vi "Handle M24.vi"(0 "reference in":refnum<class "PM_Group.lvclass">, 11 "error in (no error)":errorcluster) -> (4 "reference out":refnum<class "PM_Group.lvclass">, 15 "error out":errorcluster)   [LabVIEW 2019, in "PM_Group.lvclass"]
uses:
  PM_Group.lvclass
  C:/Users/ANENKOV_V1/Desktop/src/Device_class/Device.lvclass
  PM_Group.lvclass/PM_Group.ctl
  FPGA/TypeDef/AI index.ctl
  TypeDef/State Engine.ctl
  AI_class/AI.lvclass/AI.ctl
  AnalogComparator_class/AnalogComparator.lvclass/AnalogComparator.ctl
  Device_class/Device.lvclass/Device.ctl
  Engine_1DO_2DI_class/Engine_1DO_2DI.lvclass/Engine_1DO_2DI.ctl
  FPGA/TypeDef/DO index.ctl
  AnalogComparator_class/GetStatus.vi
  Engine_1DO_2DI_class/Engine_1DO_2DI.lvclass
  FPGA_API_class/FPGA API.lvclass
  AI_class/AI.lvclass
  Device_class/Device.lvclass
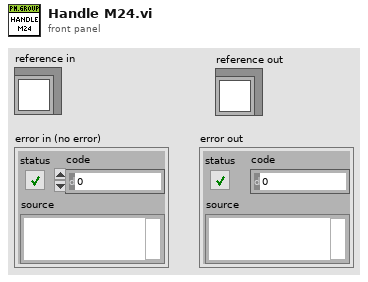
[diagram p1: front panel]
types:
  T1 = typedef "State Engine.ctl" = enum16{"Unknown", "Off", "TupningOn", "On", "TurningOff"}
  T2 = typedef "AI index.ctl" = u8
  T3 = typedef "AI_Data.ctl" = cluster{"Stat Data":T4, "OutOfRangeMax":bool, "OutOfRangeMin":bool, "HIHI":bool, "HI":bool, "LO":bool, "LOLO":bool}
  T4 = typedef "AI Statistics Data.ctl" = cluster{"raw mean":dbl, "scl mean":dbl, "raw mean 1Hz":dbl, "scl mean 1Hz":dbl}
  T5 = typedef "DO index.ctl" = u8
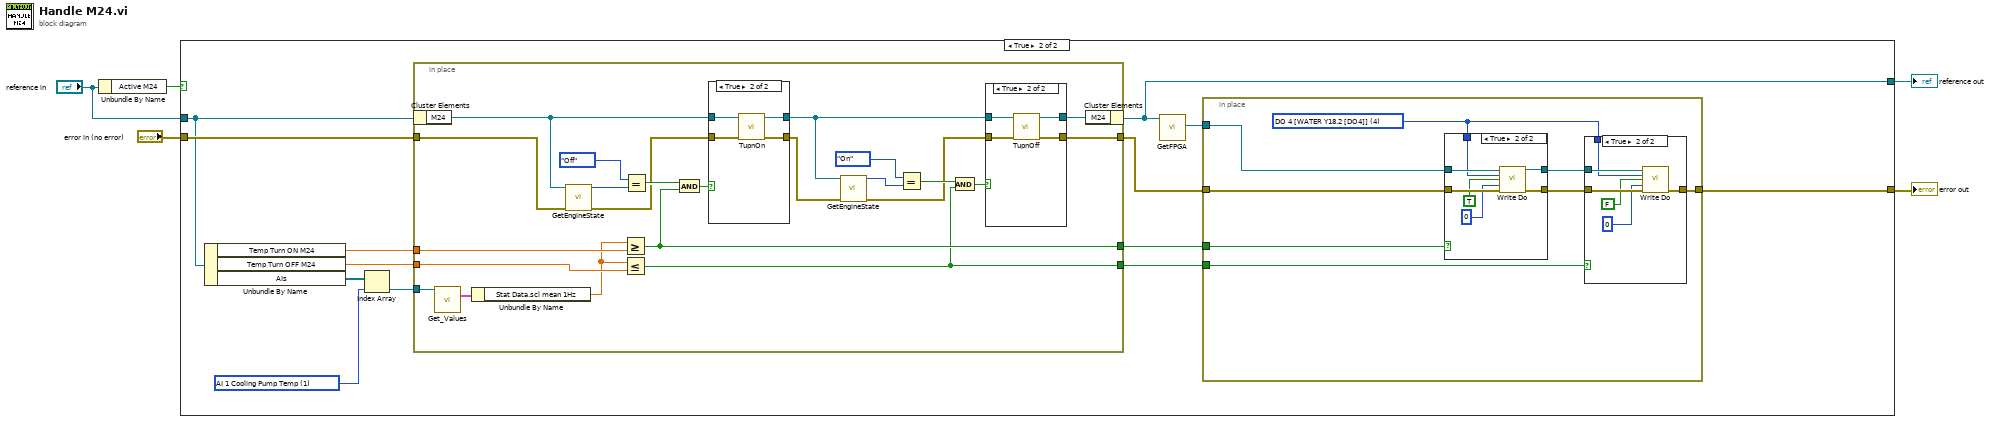
[diagram p0: block diagram]
diagram:
  n1 = Unbundle By Name("reference in") -> ("Active M24"=w1:bool)
  n2 = case shown="True" w1 {
    tunnel: "error in (no error)" -> [w6 w20]
    tunnel: "reference in" -> [w7 w14]
    tunnel: [w6 w16] -> w4
    tunnel: [w7 w15] -> w3
    frame False {
    }
    frame True {
      w10 = T2 1 items=["AI 0 Cooling Pump Level", "AI 1 Cooling Pump Temp", "AI 2 Oil Supply Level", "AI 3 Oil Supply Temp", "AI 4 ", "AI 5 Pressure Haskel", "AI 6 Pressure DUT", "AI 7 Pressure Chamber", "AI 8 Pressure Air inlet", "AI 9 Pressure Air outlet", "AI 10 Pressure Messure Line"] ("AI index")
      n3 = Unbundle By Name(w14) -> ("Temp Turn ON M24"=w13:dbl, "Temp Turn OFF M24"=w12:dbl, "AIs"=w11:refnum<class "AI.lvclass">[])
      n4 = Index Array(array=w11, index=w10) -> (element=w19:refnum<class "AI.lvclass">)
      n5 = in-place {
        in-place-border: w13 -> [w53]
        in-place-border: w12 -> [w54]
        in-place-border: w19 -> [w67]
        in-place-border: w20 -> [w50]
        in-place-border: [w59] -> w17
        in-place-border: [w46] -> w9
        in-place-border: [w45] -> w8
        n6 = in-place-cluster #1(w14) -> ("M24"=w65:refnum<class "Engine_1DO_2DI.lvclass">)
        n7 = call "Get_Values.vi"("reference in"=w67) -> ("Data"=w66:T3)  [unwired: 14 in]
        n8 = Unbundle By Name(w66) -> ("Stat Data.scl mean 1Hz"=w51:dbl)
        n9 = call "GetEngineState.vi"("Engine"=w65, "error in (no error)"=w50) -> ("EngineState"=w64:T1, "error out"=w49:errorcluster)  [unwired: 9 in, 3 out]
        n10 = Greater Or Equal?(x=w51, y=w53) -> (x >= y?=w46:bool)
        n11 = Less Or Equal?(x=w51, y=w54) -> (x <= y?=w45:bool)
        n12 = Equal?(x=State_Engine."Off" ("y"), y=w64) -> (x = y?=w62:bool)
        n13 = And(x=w62, y=w46) -> (x .and. y?=w61:bool)
        n14 = case shown="True" w61 {
          tunnel: w49 -> [w68 w73]
          tunnel: w65 -> [w69 w72]
          tunnel: [w69 w71] -> w55
          tunnel: [w68 w70] -> w48
          frame False {
          }
          frame True {
            n15 = call "TupnOn.vi"("error in (no error)"=w73, "Pump_1AI_1DO_2DI in"=w72) -> ("error out"=w70:errorcluster, "Pump_1AI_1DO_2DI out"=w71:refnum<class "Engine_1DO_2DI.lvclass">)  [unwired: 8 in]
          }
        }
        n16 = call "GetEngineState.vi"("Engine"=w55, "error in (no error)"=w48) -> ("EngineState"=w56:T1, "error out"=w47:errorcluster)  [unwired: 9 in, 3 out]
        n17 = Equal?(x=State_Engine."On" ("y"), y=w56) -> (x = y?=w58:bool)
        n18 = And(x=w58, y=w45) -> (x .and. y?=w52:bool)
        n19 = case shown="True" w52 {
          tunnel: w55 -> [w74 w79]
          tunnel: [w74 w78] -> w60
          tunnel: w47 -> [w75 w77]
          tunnel: [w75 w76] -> w59
          frame False {
          }
          frame True {
            n20 = call "TupnOff.vi"("error in (no error)"=w77, "Pump_1AI_1DO_2DI in"=w79) -> ("error out"=w76:errorcluster, "Pump_1AI_1DO_2DI out"=w78:refnum<class "Engine_1DO_2DI.lvclass">)  [unwired: 8 in]
          }
        }
        n21 = in-place-cluster #1("M24"=w60) -> (w15:refnum<class "PM_Group.lvclass">)
      }
      n22 = call "GetFPGA.vi"("Device in"=w15) -> ("FPGA API.lvclass"=w18:refnum<class "FPGA API.lvclass">)  [unwired: 10 in]
      n23 = in-place {
        in-place-border: w17 -> [w28]
        in-place-border: [w26] -> w16
        in-place-border: w18 -> [w23]
        in-place-border: w9 -> [w22]
        in-place-border: w8 -> [w21]
        w24 = T5 4 items=["DO 0 [KP1 [DO 0]]", "DO 1 [ON KP2 [DO 1]]", "DO 2 [ON KP3 [DO 2]]", "DO 3 [WATER Y18.1 [DO3]]", "DO 4 [WATER Y18.2 [DO4]]", "DO 5 [KP6 Y29.1 33.7]", "DO 6 [KP7 Y29.2 33.8]", "DO 7 [KP8 Y29.3 33.9]", "DO 8 [KP9 Y29.4  33.12]", "DO 9 [KP10 Y29.5 33.1]", "DO 10 [KP11 Y29.6 33.2]", "DO 11 [KP12 Y29.7  33.13]", "DO 12 [KP13 Y29.8  33.11]", "DO 13 [KP14 Y29.9 33.10]", "DO 14 [KP15 Y29.10  33.6]", "DO 15 [KP16 Y29.11  33.5]", "DO 16 [KP17 Y29.12  33.4]", "DO 17 [KP18 Y29.13 33.3]", "DO 18 [AIR KP19]", "DO 19 [STEP DRIVE EN KP20]", "DO 20 [KP21 Y44.1 OPEN]", "DO 21 [ KP22 Y44.1 CLOSE]", "DO 22 [ KP23 Y44.2 OPEN]", "DO 23", "DO 24 [STEP DRIVE 1]", "DO 25 [STEP DRIVE 2]"] ("#DO")
        n24 = case shown="True" w22 {
          tunnel: w28 -> [w36 w42]
          tunnel: w23 -> [w37 w44]
          tunnel: [w37 w43] -> w25
          tunnel: [w36 w41] -> w27
          tunnel: w24 -> [_ w39]
          frame False {
          }
          frame True {
            n25 = call-dynamic "Write Do.vi"("FPGA API in"=w44, "#DO"=w39, "value"=TRUE, "Time uSec"=u32 0, "error in (no error)"=w42) -> ("FPGA API out"=w43:refnum<class "FPGA API.lvclass">, "error out"=w41:errorcluster)  [unwired: 9 in]
          }
        }
        n26 = case shown="True" w21 {
          tunnel: w25 -> [_ w35]
          tunnel: w27 -> [w29 w34]
          tunnel: [w29 w33] -> w26
          tunnel: w24 -> [_ w32]
          frame False {
          }
          frame True {
            n27 = call-dynamic "Write Do.vi"("FPGA API in"=w35, "#DO"=w32, "value"=FALSE, "Time uSec"=u32 0, "error in (no error)"=w34) -> ("error out"=w33:errorcluster)  [unwired: 9 in, 1 out]
          }
        }
      }
    }
  }
  "error out" <- w4
  "reference out" <- w3
